vi "lvEtherbone.handler_getMap.vi"(0 "eb_socket_ID":i32, 1 "eb_handlerID":i32, 2 "address":u64, 3 "size":i32, 5 "error in (no error)":errorcluster) -> (13 "eb_status":T1, 14 "eb_socket_ID out":i32, 15 "eb_handlerID out":i32, 16 "data":u8[](array[numeric]), 19 "error out":errorcluster)   [LabVIEW 2009, in "lvEtherbone.lvlib"]
doc: "//-----------------------------------------------------------------------------------\n// author : Dietrich Beck, GSI-Darmstadt\n// purpose : Retrieve data from the memory map of THIS virtual device \n// by copying it from the memory map to a \"data\" buffer.\n// It is the responsibility of the caller to pre-allocate\n// sufficient memory for the data buffer prior calling this routine.\n// returns : lveb_status_t\n//-----------------------------------------------------------------------------------\nETHERBONE_API int lveb_handler_getMap( int eb_handlerID, //ID of the handler of THIS device\n eb_address_t address, //address where to read from\n int size, //size of data to read\n char *data //buffer containing read-data\n );"
uses:
  lvEtherbone.lvlib
  lvEtherbone.lveb_status_t.ctl
  bin/lvEtherbone.dll
panel:
  in  "myeb_status_t":T1
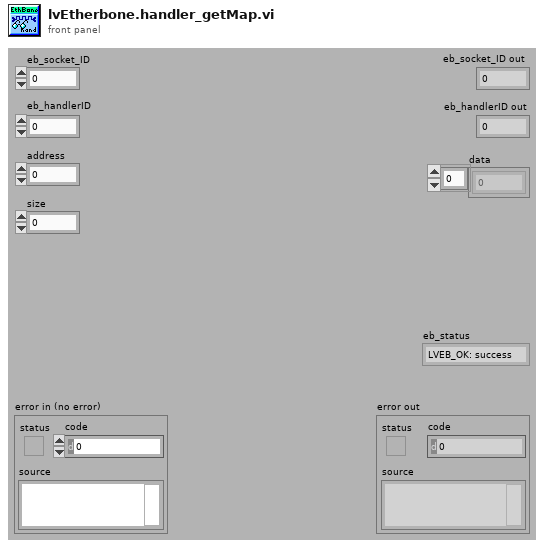
[diagram p1: front panel]
types:
  T1 = typedef "lvEtherbone.lvlib/lvEtherbone.lveb_status_t.ctl" = enum32{"LVEB_OK: success", "LVEB_UNKNOWN: unknown error", "LVEB_OS: operating system forbids access", "LVEB_PORT: port in use or unavailable", "LVEB_ID: ID invalid or out of resources", "LVEB_SOCKET: socket invalid or unavailable", "LVEB_EB: remote address is not Etherbone conformant", "LVEB_IP: bad format or network address", "LVEB_BUSWIDTH: bus width error", "LVEB_DEVICEBUSY: Whishbone device still busy", "LVEB_DEVICEFAIL: operation on Wishbone device failed", "LVEB_DEVICEEXIST: Whishbone device already exists, overlaps, or does not exist", "LVEB_TIMEDOUT: a timeout occurred", "LVEB_OVERFLOW: payload of Etherbone exceeded", "LVEB_ADDRESS: bad address"}
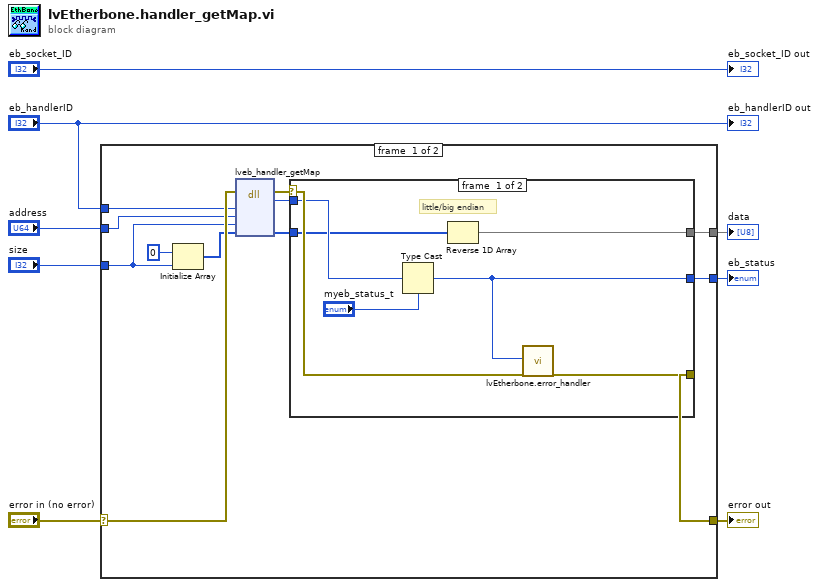
[diagram p0: block diagram]
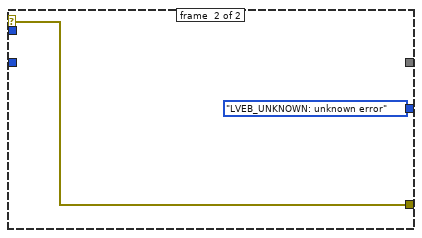
[diagram p2: hidden frame]
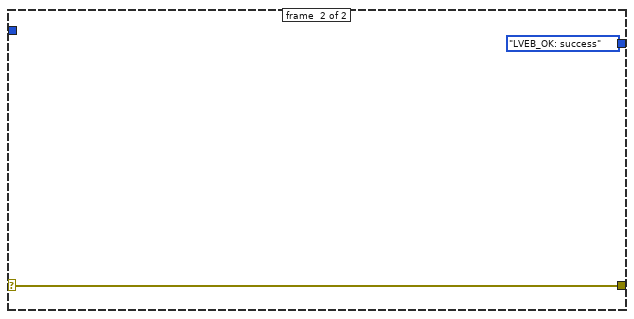
[diagram p3: hidden frame]
diagram:
  n1 = case shown="No Error" "error in (no error)" {
    selector: "error in (no error)" -> [w20 w31]
    tunnel: [w16 w31] -> w7
    tunnel: "eb_handlerID" -> [w19 _]
    tunnel: [w15 lvEtherbone.lveb_status_t."LVEB_OK: success" ("eb_status_t")] -> w6
    tunnel: "address" -> [w14 _]
    tunnel: "size" -> [w13 _]
    tunnel: [w9 _] -> w1
    frame #0 {
      n2 = Initialize Array(u8 0, w13) -> (w11:u8[])
      n3 = dll-call lib="F:/beck/Project/BEL/SCC/etherbone-core/api/lvEtherbone/bin/lvEtherbone.*" fn="lveb_handler_getMap"(error in=w20, "eb_handlersID"=w19, "address"=w14, "size"=w13, "data"=w11) -> (error out=w18:errorcluster, "myeb_status"=w17:i32, "data"=w10:u8[])  [unwired: 5 in, 1 out]
      n4 = case shown="No Error" w18 {
        selector: w18 -> [w26 w29]
        tunnel: w17 -> [w25 _]
        tunnel: [w24 lvEtherbone.lveb_status_t."LVEB_UNKNOWN: unknown error" ("eb_status_t")] -> w15
        tunnel: [w27 w29] -> w16
        tunnel: w10 -> [w22 _]
        tunnel: [w21 _] -> w9
        frame #0 {
          # "little/big endian"
          n5 = Type Cast(type="myeb_status_t", x=w25) -> (*(type *) &x=w24:T1)
          n6 = Reverse 1D Array(array=w22) -> (reversed array=w21:u8[])
          n7 = call "lvEtherbone.error_handler.vi"("eb_status"=w24, "error in"=w26) -> ("error out"=w27:errorcluster)  [unwired: 17 in]
        }
        frame #1 {
        }
      }
    }
    frame #1 {
    }
  }
  "error out" <- w7
  "eb_status" <- w6
  "data" <- w1
  "eb_socket_ID out" <- "eb_socket_ID"
  "eb_handlerID out" <- "eb_handlerID"
